vi "SEPXP Globals.vi"() -> ()   [LabVIEW 2019]
panel:
  out "Abort":bool
  in  "Phasor Explorer Version":string
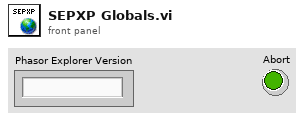
[diagram p1: front panel]
diagram:
